vi "SPI Write.vi"(9 "Write Data":u8[](array[numeric])=[0, 0, 0, 0, 0, 0, 0], 11 "Private Data In":T1) -> (2 "Read Out":u8[](array[numeric]), 3 "Private Data Out":T1)   [LabVIEW 2014]
uses:
  <vilib>/IEDriver/SPIandI2C/FPGA/Type Def/Private Data (SPI).ctl
  SPI Parameters.ctl
  <vilib>/IEDriver/SPIandI2C/FPGA/Library/IP SPI&I2C.lvlib
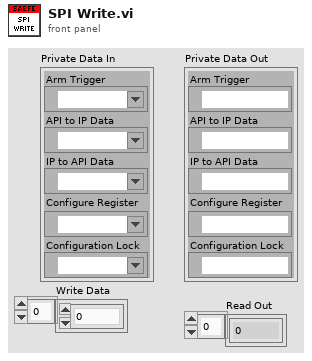
[diagram p1: front panel]
types:
  T1 = typedef "IP SPI&I2C.lvlib/Private Data (SPI).ctl" = cluster{"Arm Trigger":refnum<k21>, "API to IP Data":refnum<k21>, "IP to API Data":refnum<k21>, "Configure Register":refnum<k21>, "Configuration Lock":refnum<k21>}
  T2 = typedef "SPI Parameters.ctl" = cluster{"Clock Divider":u32, "Mode":u8, "CS Active State":bool}
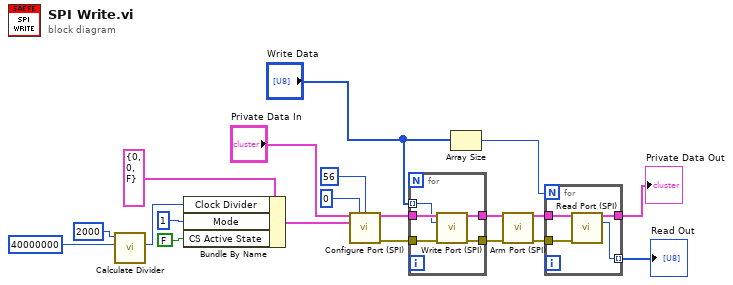
[diagram p0: block diagram]
diagram:
  n1 = call <vilib>:"Calculate Divider.vi"("FPGA Clock (Hz)"=u32 40000000 ("Clock Rate (Hz)"), "Clock Rate (Hz)"=u32 2000) -> ("Clock Divider"=w17:u32)  [unwired: 7 in, 2 out]
  n2 = Bundle By Name(cluster=T2 {"Clock Divider"=0, "Mode"=0, "CS Active State"=FALSE} ("SPI Parameters"), "Clock Divider"=w17, "Mode"=u8 1, "CS Active State"=FALSE) -> (w15:T2)
  n3 = call <vilib>:"Configure Port (SPI).vi"("Private Data In"="Private Data In", "Chip Select"=u8 0, "Number of Bits"=u16 56, "SPI Parameters"=w15) -> ("Private Data Out"=w11:T1, "error out"=w10:errorcluster)  [unwired: 9 in, 1 out]
  n4 = for {
    tunnel: "Write Data" -> [w21] mode=indexing
    tunnel: w11 -> [w25]
    tunnel: [w23] -> w7
    tunnel: w10 -> [w24]
    tunnel: [w22] -> w6
    n5 = call <vilib>:"Write Port (SPI).vi"("Private Data In"=w25, "Data In"=w21, "error in"=w24) -> ("Private Data Out"=w23:T1, "error out"=w22:errorcluster)  [unwired: 10 in, 1 out]
  }
  n6 = Array Size(array="Write Data") -> (size(s)=w1:i32)
  n7 = call <vilib>:"Arm Port (SPI).vi"("Private Data In"=w7, "error in"=w6) -> ("Private Data Out"=w5:T1, "error out"=w4:errorcluster)  [unwired: 11 in, 1 out]
  n8 = for {
    N: w1 -> [_]
    tunnel: w5 -> [w29]
    tunnel: w4 -> [w28]
    tunnel: [w27] -> w3 mode=indexing
    tunnel: [w26] -> w20
    n9 = call <vilib>:"Read Port (SPI).vi"("Private Data In"=w29, "error in"=w28) -> ("Private Data Out"=w26:T1, "Data Out"=w27:u8)  [unwired: 10 in, 2 out]
  }
  "Private Data Out" <- w20
  "Read Out" <- w3
